vi "Extract Vibratome.vi"(10 "Vibratome Controls":T2, 11 "Vibratome":T1) -> (3 "Vibratome Out":T1)   [LabVIEW 2018]
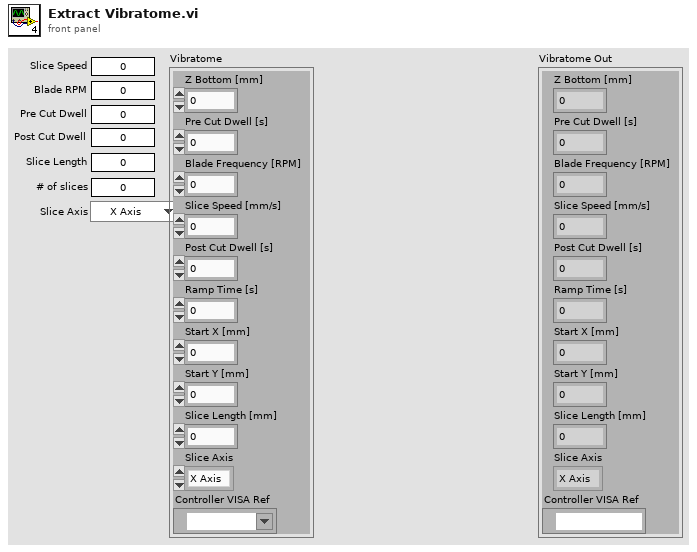
[diagram p1: front panel]
types:
  T1 = cluster{"Z Bottom [mm]":dbl, "Pre Cut Dwell [s]":dbl, "Blade Frequency [RPM]":u16, "Slice Speed [mm/s]":dbl, "Post Cut Dwell [s]":dbl, "Ramp Time [s]":dbl, "Start X [mm]":dbl, "Start Y [mm]":dbl, "Slice Length [mm]":dbl, "Slice Axis":enum16{"X Axis", "Y Axis", "Z Axis"}, "Controller VISA Ref":refnum<visa-resource-name>}
  T2 = cluster{"Pre Cut Dwell":dbl, "Blade RPM":u16, "Slice Speed":dbl, "Post Cut Dwell":dbl, "Slice Length":dbl, "# of slices":dbl, "Slice Axis":enum16{"X Axis", "Y Axis", "Z Axis"}}
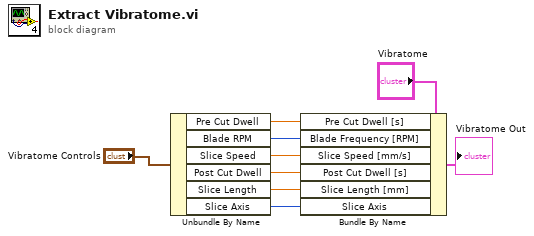
[diagram p0: block diagram]
diagram:
  n1 = Unbundle By Name("Vibratome Controls") -> ("Pre Cut Dwell"=w7:dbl, "Blade RPM"=w6:u16, "Slice Speed"=w5:dbl, "Post Cut Dwell"=w4:dbl, "Slice Length"=w3:dbl, "Slice Axis"=w1:enum16{"X Axis", "Y Axis", "Z Axis"})
  n2 = Bundle By Name(cluster="Vibratome", "Pre Cut Dwell [s]"=w7, "Blade Frequency [RPM]"=w6, "Slice Speed [mm/s]"=w5, "Post Cut Dwell [s]"=w4, "Slice Length [mm]"=w3, "Slice Axis"=w1) -> (→"Vibratome Out":T1)
